vi "Get Variables.vi"(8 "error in (no error)":errorcluster, 11 "Message Popup in":refnum<class "Array Functions.lvclass">) -> (0 "error out":errorcluster, 2 "Variables":variant, 3 "Message Popup out":refnum<class "Array Functions.lvclass">)   [LabVIEW 2019, in "Array Functions.lvclass"]
uses:
  Array Functions.lvclass
  Array Functions.lvclass/Array Functions.ctl
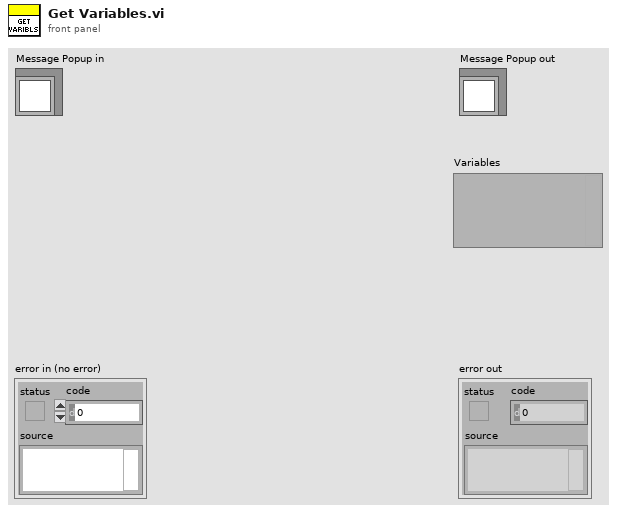
[diagram p1: front panel]
types:
  T1 = typedef "Array Functions.lvclass/Variables.ctl" = cluster{"Var1":variant, "Var2":variant, "Index1":i32, "Index2":i32, "Length1":i32, "Length2":i32, "leftoperand":string}
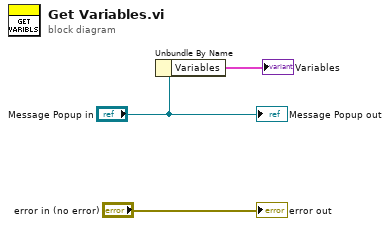
[diagram p0: block diagram]
diagram:
  n1 = Unbundle By Name("Message Popup in") -> ("Variables"=→"Variables":T1)
  "error out" <- "error in (no error)"
  "Message Popup out" <- "Message Popup in"
